vi "Test Strict Ambiguous ISO8601 Strings.vi"(8 "error in (no error)":errorcluster) -> (0 "error out":errorcluster)   [LabVIEW 2017]
uses:
  <vilib>/Utility/file.llb/Read From Spreadsheet File (string).vi
  <vilib>/addons/_JKI Toolkits/Caraya/classes/Assert/Assert False.vi
  <vilib>/addons/_JKI Toolkits/Caraya/classes/Assert/Assert True.vi
  <vilib>/addons/_JKI Toolkits/Caraya/classes/Assert/Assert.lvclass
  <vilib>/addons/_JKI Toolkits/Caraya/classes/Test/Test.lvclass
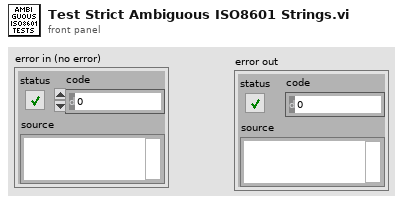
[diagram p1: front panel]
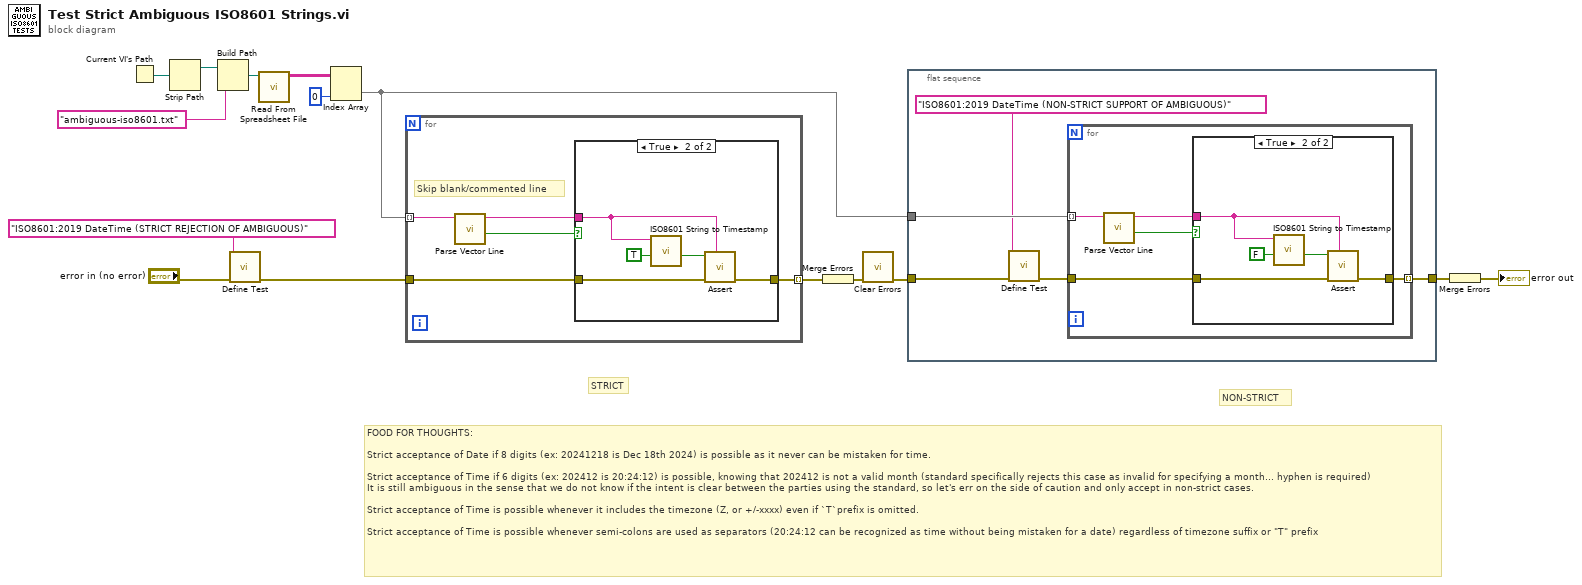
[diagram p0: block diagram]
diagram:
  # "NON-STRICT"
  # "STRICT"
  # "FOOD FOR THOUGHTS:\n\nStrict acceptance of Date if 8 digits (ex: 20241218 is Dec 18th 2024) is possible as it never can be mistaken for time.\n\nStrict acceptance of Time if 6 digits (ex: 202412 is 20:24:12) is possible, knowing that 202412 is not a valid month (standard specifically rejects this case as invalid for specifying a month... hyphen is required)\nIt is still ambiguous in the sense that we do not know if the intent is clear between the parties using the standard, so let's err on the side of caution and only accept in non-strict cases.\n\nStrict acceptance of Time is possible whenever it includes the timezone (Z, or +/-xxxx) even if `T`prefix is omitted.\n\nStrict acceptance of Time is possible whenever semi-colons are used as separators (20:24:12 can be recognized as time without being mistaken for a date) regardless of timezone suffix or \"T\" prefix"
  n1 = Current VI's Path() -> (path=w9:path)
  n2 = Strip Path(path=w9) -> (stripped path=w10:path)  [unwired: 1 out]
  n3 = Build Path(base path=w10, name or relative path="ambiguous-iso8601.txt") -> (appended path=w11:path)
  n4 = call <vilib>:"Define Test.vi"("error in (no error)"="error in (no error)", "Label (VI Title)"="ISO8601:2019 DateTime (STRICT REJECTION OF AMBIGUOUS)") -> ("error out"=w14:errorcluster)  [unwired: 8 in, 1 out]
  n5 = call-poly <vilib>:"Read From Spreadsheet File.vi"("file path (dialog if empty)"=w11) -> ("all rows"=w7:string[][])  [unwired: 6 in, 4 out]
  n6 = Index Array(array=w7, index (col)=0 ("disabled index (col)")) -> (element=w3:string[])  [unwired: 1 in]
  n7 = for {
    tunnel: w3 -> [w18] mode=indexing
    tunnel: [w19] -> w5 mode=indexing
    tunnel: w14 -> [w20]
    # "Skip blank/commented line"
    n8 = call "Parse Vector Line.vi"("string"=w18) -> ("perform test"=w16:bool, "string out"=w17:string)  [unwired: 9 in]
    n9 = case shown="True" w16 {
      tunnel: w20 -> [w21 w26]
      tunnel: [w21 w25] -> w19
      tunnel: w17 -> [_ w22]
      frame False {
        # "Skip"
      }
      frame True {
        n10 = call "ISO8601 String to Timestamp.vi"("Strict ISO? (T)"=TRUE, "ISO8601 String"=w22) -> ("valid?"=w23:bool)  [unwired: 7 in, 2 out]
        n11 = call-poly <vilib>:"Assert.vi"("Label"=w22, "error in (no error)"=w26, "False?"=w23) -> ("error out"=w25:errorcluster)  [unwired: 7 in, 1 out]
      }
    }
  }
  n12 = Merge Errors(w5) -> (w4:errorcluster)
  n13 = call <vilib>:"Clear Errors.vi"("error in (no error)"=w4) -> ("error out"=w1:errorcluster)  [unwired: 5 in, 1 out]
  n14 = flat-sequence {
    tunnel: w3 -> [w31]
    tunnel: [w30] -> w2
    tunnel: w1 -> [w28]
    frame #0 {
      n15 = call <vilib>:"Define Test.vi"("error in (no error)"=w28, "Label (VI Title)"="ISO8601:2019 DateTime (NON-STRICT SUPPORT OF AMBIGUOUS)") -> ("error out"=w27:errorcluster)  [unwired: 8 in, 1 out]
      n16 = for {
        tunnel: w31 -> [w34] mode=indexing
        tunnel: [w35] -> w30 mode=indexing
        tunnel: w27 -> [w36]
        n17 = call "Parse Vector Line.vi"("string"=w34) -> ("perform test"=w32:bool, "string out"=w33:string)  [unwired: 9 in]
        n18 = case shown="True" w32 {
          tunnel: w36 -> [w37 w42]
          tunnel: [w37 w41] -> w35
          tunnel: w33 -> [_ w38]
          frame False {
            # "Skip"
          }
          frame True {
            n19 = call "ISO8601 String to Timestamp.vi"("Strict ISO? (T)"=FALSE, "ISO8601 String"=w38) -> ("valid?"=w39:bool)  [unwired: 7 in, 2 out]
            n20 = call-poly <vilib>:"Assert.vi"("Label"=w38, "error in (no error)"=w42, "True?"=w39) -> ("error out"=w41:errorcluster)  [unwired: 7 in, 1 out]
          }
        }
      }
    }
  }
  n21 = Merge Errors(w2) -> (→"error out":errorcluster)
